vi "Get_SLOPE_data_from_file 2016.vi"(11 "Slopes File Path":path=path "D:/Cascade/Data/Output Files/slopes.txt") -> (0 "Last_Pressure_Slope":dbl format="%.2f", 1 "Last_Flow_Slope":dbl format="%.2f", 2 "Last_String_Pot_Slope":dbl format="%.2f", 3 "Output_array":sgl[][](array[numeric]) format="%.2f")   [LabVIEW 2016]
uses:
  <vilib>/Utility/file.llb/Read Delimited Spreadsheet (DBL).vi
  <vilib>/Utility/file.llb/Read Delimited Spreadsheet (string).vi
panel:
  out "number of rows\n(including header)":i32
  out "first row":string[][](array[string])
  out "file or folder exists?":bool
  out "error out":errorcluster
  out "Last_KPRO_Box_Number":dbl
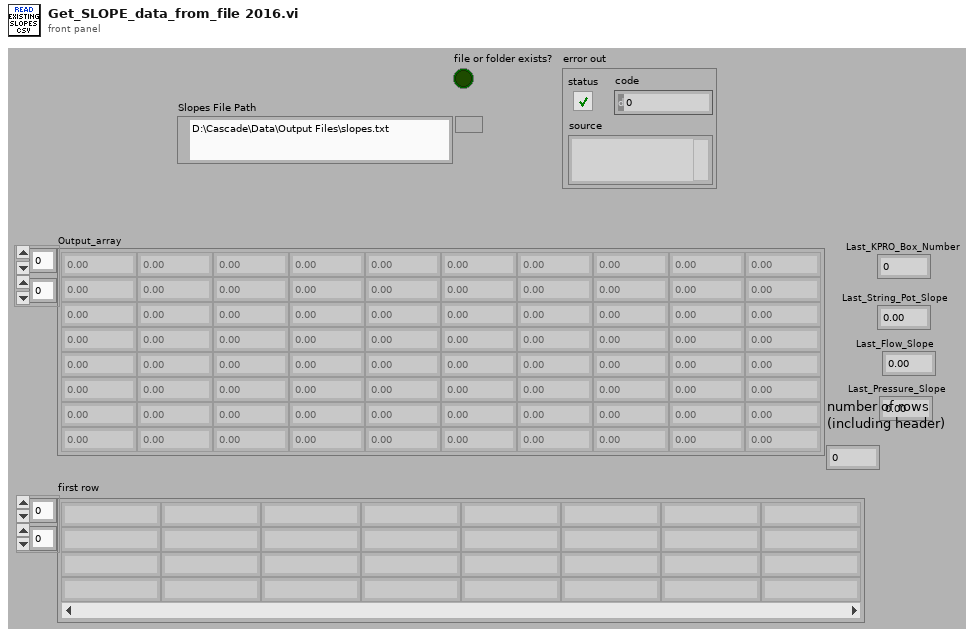
[diagram p1: front panel]
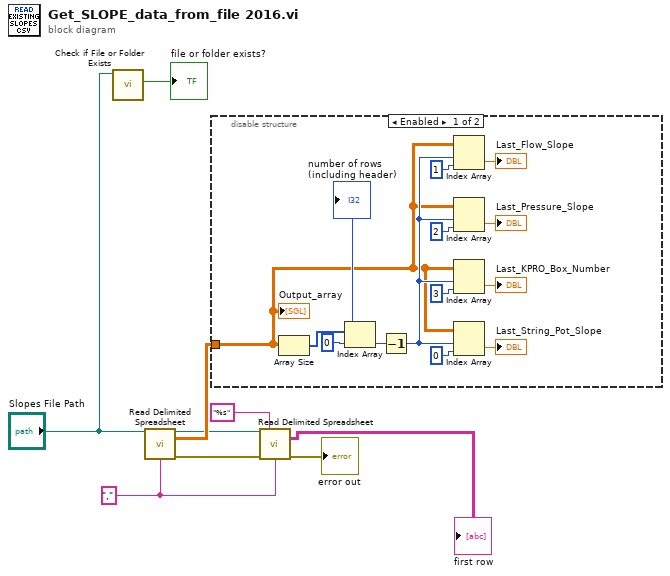
[diagram p0: block diagram]
diagram:
  w1 = ","
  n1 = call <vilib>:"Check if File or Folder Exists.vi"("path"="Slopes File Path") -> ("file or folder exists?"=→"file or folder exists?":bool)  [unwired: 8 in, 2 out]
  n2 = call-poly <vilib>:"Read Delimited Spreadsheet.vi"("file path (dialog if empty)"="Slopes File Path", "delimiter (\\t)"=w1) -> ("new file path (Not A Path if cancelled)"=w6:path, "all rows"=w9:dbl[][], "error out"=w4:errorcluster)  [unwired: 8 in, 3 out]
  n3 = disable-structure shown="Enabled" {
    disable-tunnel: w9 -> [w10 _]
    frame Enabled {
      n4 = Array Size(array=w10) -> (size(s)=w21:i32[])
      n5 = Index Array(array=w21, index=0) -> (element=w20:i32)
      "number of rows\n(including header)" <- w20
      n6 = Decrement(x=w20) -> (x-1=w13:i32)
      n7 = Index Array(array=w10, index (row)=w13, index (col)=1 ("disabled index (col)")) -> (element=→"Last_Flow_Slope":dbl)
      n8 = Index Array(array=w10, index (row)=w13, index (col)=2 ("index")) -> (element=→"Last_Pressure_Slope":dbl)
      n9 = Index Array(array=w10, index (row)=w13, index (col)=3 ("index")) -> (element=→"Last_KPRO_Box_Number":dbl)
      n10 = Index Array(array=w10, index (row)=w13, index (col)=0 ("index")) -> (element=→"Last_String_Pot_Slope":dbl)
      "Output_array" <- w10
    }
    frame Disabled {
    }
  }
  n11 = call-poly <vilib>:"Read Delimited Spreadsheet.vi"("file path (dialog if empty)"=w6, "format (%s)"="%s" ("format (%.3f)"), "error in (no error)"=w4, "delimiter (\\t)"=w1) -> ("all rows"=→"first row":string[][], "error out"=→"error out":errorcluster)  [unwired: 6 in, 4 out]
